vi "Global 1.vi"() -> ()   [LabVIEW 2014]
panel:
  out "drone index":i32
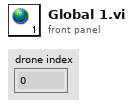
[diagram p1: front panel]
diagram:
